vi "Main.vi"(11 "Module Admin":refnum<class "Delacor_lib_QMH_Cloneable Module Admin.lvclass">) -> ()   [LabVIEW 2023, in "Graph_data_collector.lvlib" / "Graph_UI.lvlib"]
doc: "This template is based off of the Queued Message Handler design pattern and the Queued Message Handler project template that ships with LabVIEW.\n\nThe main difference is that the queue is private to this module and communication between modules is performed via Broadcast and Request events.\n\nRequest events are wrapped in public API methods and are handled in the Event Handling Loop (EHL) of this VI. Any module can register for Broadcast events sent by this module. The EHL generates messages based on user interface actions.\n\nThe Message Handling Loop (MHL) processes messages generated by the EHL, or by other messages. The messages are string values, so new messages can be added easily to the Message Cases case structure in the MHL. Each message cluster can also provide an optional value for Message Data, which is a variant that can be converted to whatever message-specific data is required.\n_____\nBased on DQMH Project Template 6.1.0.94."
uses:
  Graph_UI.lvlib
  <vilib>/Delacor/Delacor QMH/Libraries/Cloneable Module Admin_class/Delacor_lib_QMH_Cloneable Module Admin.lvclass
  C:/Program Files/National Instruments/LabVIEW 2023/vi.lib/Delacor/Delacor QMH/Libraries/Module Admin_class/Delacor_lib_QMH_Module Admin.lvclass
  Module Data--cluster.ctl
  Data Control.ctl
  <vilib>/Delacor/Delacor QMH/Libraries/Message Queue_class/Delacor_lib_QMH_Message Queue.lvclass/Delacor_lib_QMH_Message Queue.ctl
  <vilib>/Delacor/Delacor QMH/Libraries/Cloneable Module Admin_class/Delacor_lib_QMH_Cloneable Module Admin.lvclass/Delacor_lib_QMH_Cloneable Module Admin.ctl
  Stop Argument--cluster.ctl
  New Data Argument--cluster.ctl
  SetP Argument--cluster.ctl
  <vilib>/Utility/miscctls.llb/LVPointTypeDef.ctl
  <vilib>/Delacor/Delacor QMH/Libraries/Module Admin_class/Delacor_lib_QMH_Module Admin.lvclass/Delacor_lib_QMH_Module Admin.ctl
  <vilib>/Delacor/Delacor QMH/Libraries/Message Queue_class/Delacor_lib_QMH_Enqueue Message (Single).vi
  <vilib>/Delacor/Delacor QMH/Libraries/Cloneable Module Admin_class/Delacor_lib_QMH_Get Module ID.vi
  <vilib>/Delacor/Delacor QMH/Libraries/Module Admin_class/Delacor_lib_QMH_Get External Launch.vi
  <vilib>/Utility/error.llb/Error Cluster From Error Code.vi
  <vilib>/ErrorRing/Error Ring.xnode
  <vilib>/Delacor/Delacor QMH/Libraries/Message Queue_class/Delacor_lib_QMH_Message Queue.lvclass
  Graph_data_collector.lvlib
panel:
  out "Общая ось":bool
  out "Персональные оси":bool
  in  "Оси":bool
  in  "Clear_Graph":bool
  out "error out":errorcluster
  out "Status":string
  in  "Simulate EHL Error":bool
  in  "Simulate MHL Error":bool
  out "XY Graph Time":cluster{"Value":timestamp[], "Value":dbl[]}[](graph)
  out "XY Graph Other":cluster{"OX":dbl[], "OY":dbl[]}[](graph)
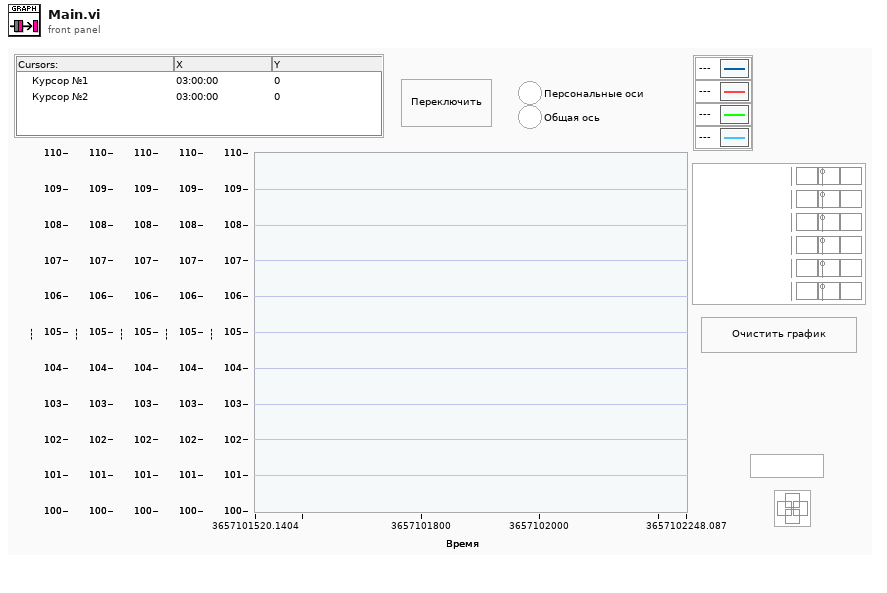
[diagram p1: front panel]
types:
  T1 = typedef "Graph_data_collector.lvlib/Graph_UI.lvlib/Module Data--cluster.ctl" = cluster{"Status":string, "XY Graph our ref":refnum<vi>, "Array Lable":string[], "Ось Y":i32[], "Ось Х":i32, "Graph size":i32, "appended array":T2[], "XY Graph ref":refnum<vi>}
  T2 = typedef "Graph_data_collector.lvlib/Data Control.ctl" = cluster{"Время":dbl, "Рпл1, МПа":dbl, "Vпл, см3":dbl, "Рпл2, МПа":dbl, "Ргор, МПа":dbl, "Ткд, градС":dbl, "R, Ом":dbl, "dL, мм":dbl, "Рэфф, МПа":dbl, "Рдм, МПа":dbl, "Q, мл":dbl, "Тнагр, градС":dbl, "ЦАП, градС":dbl}
  T3 = typedef "Graph_data_collector.lvlib/Graph_UI.lvlib/Request Events--cluster.ctl" = cluster{"Stop Module":refnum<user-event>, "Show Panel":refnum<user-event>, "Hide Panel":refnum<user-event>, "Show Diagram":refnum<user-event>, "Get Module Execution Status":refnum<user-event>, "New Data":refnum<user-event>, "SetP":refnum<user-event>}
  T4 = enum32{"invalid lock state", "Not Locked", "Locked (No Password)", "Password-protected"}
  T5 = typedef "Graph_data_collector.lvlib/Graph_UI.lvlib/Stop Argument--cluster.ctl" = cluster{"Module ID":i32, "Origin":string, "Exit via Stop Module Req?":bool, "Wait for Module to stop?":bool}
  T6 = typedef "Graph_data_collector.lvlib/Graph_UI.lvlib/New Data Argument--cluster.ctl" = cluster{"Module ID":i32, "Data":T2}
  T7 = typedef "Graph_data_collector.lvlib/Graph_UI.lvlib/SetP Argument--cluster.ctl" = cluster{"Module ID":i32, "Module Data":T1}
  T8 = typedef "LVPointTypeDef.ctl" = cluster{"Horizontal":i16, "Vertical":i16}
  T9 = enum32{"Invalid", "Standard", "Closed", "Hidden", "Minimized", "Maximized"}
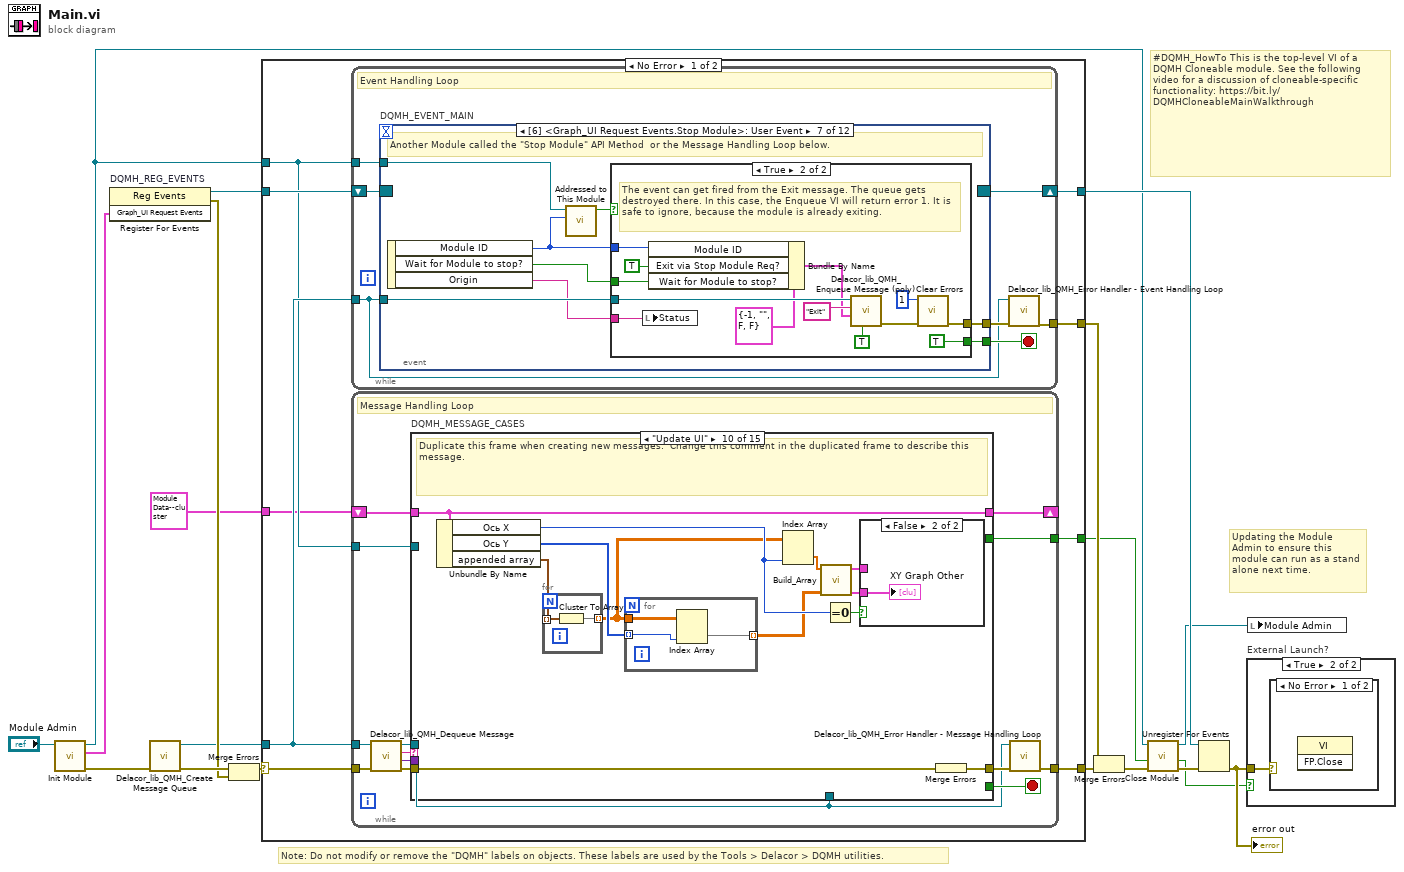
[diagram p0: block diagram]
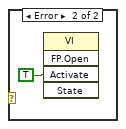
[diagram p3: hidden frame]
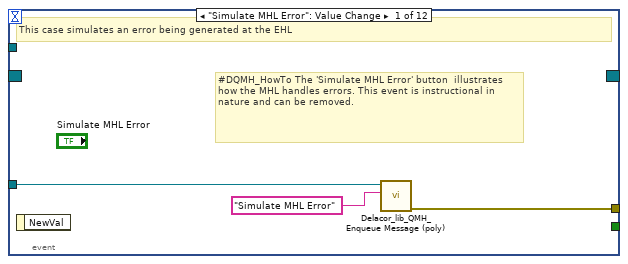
[diagram p4: hidden frame]
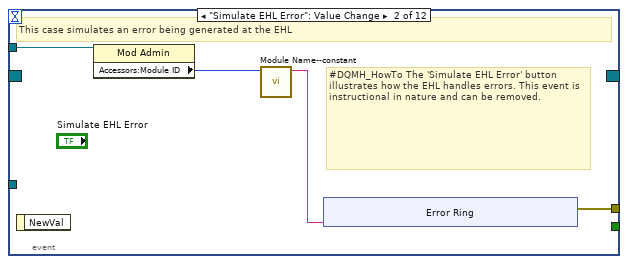
[diagram p5: hidden frame]
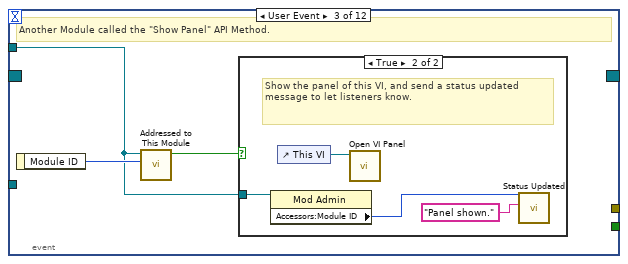
[diagram p6: hidden frame]
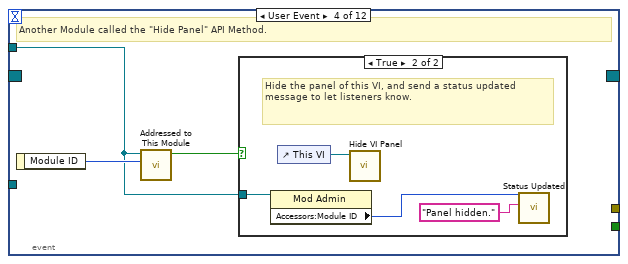
[diagram p8: hidden frame]
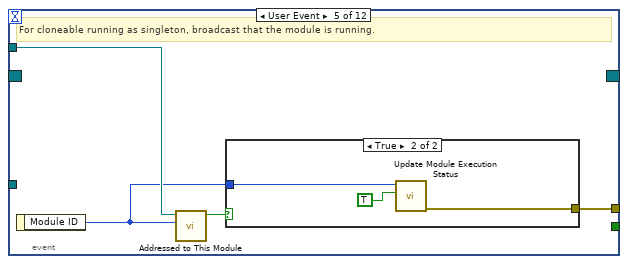
[diagram p10: hidden frame]
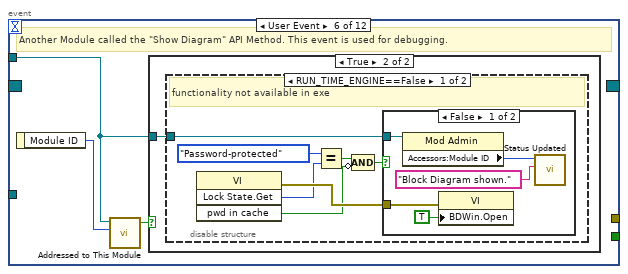
[diagram p12: hidden frame]
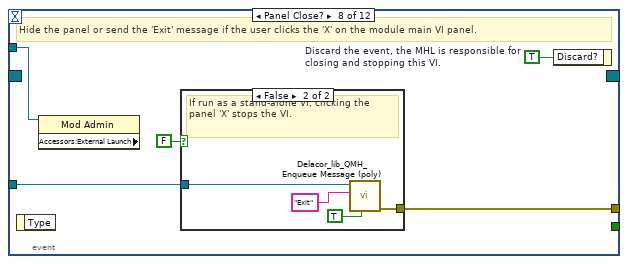
[diagram p17: hidden frame]
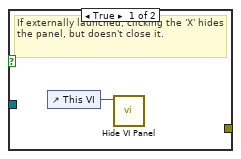
[diagram p18: hidden frame]
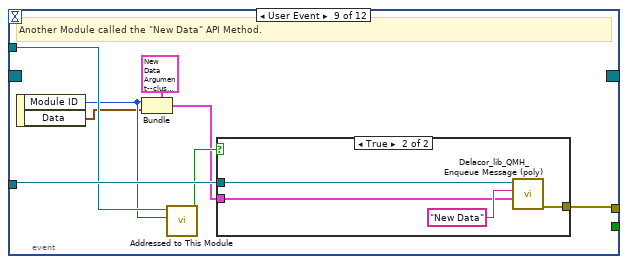
[diagram p19: hidden frame]
diagram:
  # "#DQMH_HowTo This is the top-level VI of a DQMH Cloneable module. See the following video for a discussion of cloneable-specific functionality: https://bit.ly/DQMHCloneableMainWalkthrough"
  # "Note: Do not modify or remove the \"DQMH\" labels on objects. These labels are used by the Tools > Delacor > DQMH utilities."
  # "Updating the Module Admin to ensure this module can run as a stand alone next time."
  n1 = call "Init Module.vi"("Cloneable Module Admin in"="Module Admin") -> ("error out"=w16:errorcluster, "Graph_UI Request Events"=w8:T3, "Cloneable Module Admin out"=w5:refnum<class "Delacor_lib_QMH_Cloneable Module Admin.lvclass">)  [unwired: 8 in]
  n2 = register-events "DQMH_REG_EVENTS"(w8) -> (reference out=w9:refnum<event-registration>, error out=w11:errorcluster)  [unwired: 2 in]
  n3 = call <vilib>:"Delacor_lib_QMH_Create Message Queue.vi"("error in"=w16) -> ("error out"=w13:errorcluster, "Message Queue"=w7:refnum<class "Delacor_lib_QMH_Message Queue.lvclass">)  [unwired: 9 in]
  n4 = Merge Errors(w13, w11) -> (w12:errorcluster)
  n5 = case shown="No Error" w12 {
    selector: w12 -> [w26 w356]
    tunnel: [w28 w355] -> w17
    tunnel: [w25 w363] -> w10
    tunnel: w9 -> [w24 w363]
    tunnel: w7 -> [w23 w354]
    tunnel: [w27 _] -> w18
    tunnel: w5 -> [w22 w359]
    tunnel: [w21 _] -> w3
    tunnel: T1 {"Status"="", "XY Graph our ref"=refnum, "Array Lable"=[], "Ось Y"=[], "Ось Х"=0, "Graph size"=20000, "appended array"=[], "XY Graph ref"=refnum} ("Data Cluster") -> [w20 _]
    frame No Error {
      n6 = while {
        tunnel: w23 -> [w29]
        shift-right: [w32] -> w25
        shift-left: w24 -> [w33]
        tunnel: [w34] -> w27
        tunnel: w22 -> [w30]
        stop <- w31 stop-if-true
        # "Event Handling Loop"
        n7 = event "DQMH_EVENT_MAIN" shown="[6] <Graph_UI Request Events.Stop Module>: User Event" {
          selector: w33 -> [_ _ _ _ _ _ _ _ _ _ _ _]
          dyn-events: [_ _ _ _ _ _ _ _ _ _ _ _] -> w32
          timeout: _ -> [_ _ _ _ _ _ _ _ _ _ _ _]
          tunnel: [_ _ _ _ _ _ w90 _ _ _ _ _] -> w31
          tunnel: w29 -> [w37 _ _ _ _ _ w93 w109 w125 w131 w140 w146]
          tunnel: [w38 w42 _ _ w67 _ w94 w112 w118 w130 w133 w145] -> w35
          tunnel: w30 -> [_ w41 w50 w57 w65 w71 w92 w110 w123 _ w138 _]
          event "Simulate MHL Error": Value Change {
            # "#DQMH_HowTo The 'Simulate MHL Error' button  illustrates how the MHL handles errors. This event is instructional in nature and can be removed."
            # "This case simulates an error being generated at the EHL"
            n8 = event-data() -> ()  [unwired: 1 in, 1 out]
            n9 = call-poly <vilib>:"Delacor_lib_QMH_Enqueue Message (poly).vi"("Message"="Simulate MHL Error", "Message Queue in"=w37) -> ("error out"=w38:errorcluster)  [unwired: 8 in, 1 out]
          }
          event "Simulate EHL Error": Value Change {
            # "#DQMH_HowTo The 'Simulate EHL Error' button  illustrates how the EHL handles errors. This event is instructional in nature and can be removed."
            # "This case simulates an error being generated at the EHL"
            n10 = event-data() -> ()  [unwired: 1 in, 1 out]
            n11 = property class="Mod Admin"(reference=w41) -> ("Accessors:Module ID"=w40:i32)  [unwired: 1 in, 2 out]
            n12 = call "Module Name--constant.vi"("Module ID"=w40) -> ("Module Name"=w39:string)  [unwired: 10 in]
            n13 = xnode "Error Ring"("parameter 0"=w39) -> ("error out"=w42:errorcluster)
          }
          event User Event {
            # "Another Module called the \"Show Panel\" API Method."
            n14 = event-data() -> ("Module ID"=w51:i32)  [unwired: 1 in]
            n15 = call "Addressed to This Module.vi"("Module ID from Argument"=w51, "Module Admin"=w50) -> ("Addressed to this instance?"=w52:bool)  [unwired: 8 in, 1 out]
            n16 = case shown="True" w52 {
              tunnel: w50 -> [_ w54]
              frame False {
              }
              frame True {
                # "Show the panel of this VI, and send a status updated message to let listeners know."
                n17 = property class="Mod Admin"(reference=w54) -> ("Accessors:Module ID"=w53:i32)  [unwired: 1 in, 2 out]
                n18 = control-ref of="This VI"() -> (w56:refnum<vi>)
                n19 = call "Open VI Panel.vi"("VI"=w56) -> ()  [unwired: 10 in, 1 out]
                n20 = call "Status Updated.vi"("Status"="Panel shown." ("format string"), "Module ID"=w53) -> ()  [unwired: 9 in, 1 out]
              }
            }
          }
          event User Event {
            # "Another Module called the \"Hide Panel\" API Method."
            n21 = event-data() -> ("Module ID"=w58:i32)  [unwired: 1 in]
            n22 = call "Addressed to This Module.vi"("Module ID from Argument"=w58, "Module Admin"=w57) -> ("Addressed to this instance?"=w59:bool)  [unwired: 8 in, 1 out]
            n23 = case shown="True" w59 {
              tunnel: w57 -> [_ w61]
              frame False {
              }
              frame True {
                # "Hide the panel of this VI, and send a status updated message to let listeners know."
                n24 = property class="Mod Admin"(reference=w61) -> ("Accessors:Module ID"=w60:i32)  [unwired: 1 in, 2 out]
                n25 = control-ref of="This VI"() -> (w63:refnum<vi>)
                n26 = call "Hide VI Panel.vi"("VI"=w63) -> ()  [unwired: 10 in, 1 out]
                n27 = call "Status Updated.vi"("Status"="Panel hidden." ("format string"), "Module ID"=w60) -> ()  [unwired: 9 in, 1 out]
              }
            }
          }
          event User Event {
            # "For cloneable running as singleton, broadcast that the module is running."
            n28 = event-data() -> ("Module ID"=w64:i32)  [unwired: 1 in]
            n29 = call "Addressed to This Module.vi"("Module ID from Argument"=w64, "Module Admin"=w65) -> ("Addressed to this instance?"=w66:bool)  [unwired: 8 in, 1 out]
            n30 = case shown="True" w66 {
              tunnel: [_ w70] -> w67
              tunnel: w64 -> [_ w69]
              frame False {
              }
              frame True {
                n31 = call "Update Module Execution Status.vi"("Running?"=TRUE, "Module ID"=w69) -> ("error out"=w70:errorcluster)  [unwired: 9 in]
              }
            }
          }
          event User Event {
            # "Another Module called the \"Show Diagram\" API Method. This event is used for debugging."
            n32 = event-data() -> ("Module ID"=w72:i32)  [unwired: 1 in]
            n33 = call "Addressed to This Module.vi"("Module ID from Argument"=w72, "Module Admin"=w71) -> ("Addressed to this instance?"=w73:bool)  [unwired: 8 in, 1 out]
            n34 = case shown="True" w73 {
              tunnel: w71 -> [_ w74]
              frame False {
              }
              frame True {
                n35 = disable-structure shown="RUN_TIME_ENGINE==False" {
                  disable-tunnel: w74 -> [w75 _]
                  frame condition #0 (active) {
                    # "functionality not available in exe"
                    n36 = invoke class="VI" method="Lock State.Get"() -> (error out=w81:errorcluster, "Get Lock State"=w80:T4, "pwd in cache"=w77:bool)  [unwired: 4 in, 1 out]
                    n37 = Equal?(x=T4."Password-protected", y=w80) -> (x = y?=w78:bool)
                    n38 = Compound Arithmetic op=AND(w78, invert w77) -> (w76:bool)
                    n39 = case shown="False" w76 {
                      tunnel: w81 -> [w86 _]
                      tunnel: w75 -> [w83 _]
                      frame False {
                        n40 = property class="Mod Admin"(reference=w83) -> ("Accessors:Module ID"=w82:i32)  [unwired: 1 in, 2 out]
                        n41 = property class="VI"(error in=w86, "BDWin.Open"=TRUE ("Block Diagram Window:Open")) -> ()  [unwired: 1 in, 2 out]
                        n42 = call "Status Updated.vi"("Status"="Block Diagram shown." ("format string"), "Module ID"=w82) -> ()  [unwired: 9 in, 1 out]
                      }
                      frame True {
                        # "Password-protected VI, and the password is not in the cache. Do not show the diagram."
                      }
                    }
                  }
                  frame condition #1 {
                  }
                }
              }
            }
          }
          event User Event {
            # "Another Module called the \"Stop Module\" API Method  or the Message Handling Loop below."
            n43 = event-data() -> ("Module ID"=w88:i32, "Wait for Module to stop?"=w89:bool, "Origin"=w87:string)  [unwired: 1 in]
            n44 = call "Addressed to This Module.vi"("Module ID from Argument"=w88, "Module Admin"=w92) -> ("Addressed to this instance?"=w91:bool)  [unwired: 8 in, 1 out]
            n45 = case shown="True" w91 {
              tunnel: [_ w106] -> w94
              tunnel: w93 -> [_ w102]
              tunnel: [_ TRUE] -> w90
              tunnel: w89 -> [_ w97]
              tunnel: w88 -> [_ w99]
              tunnel: w87 -> [_ w95]
              frame False {
              }
              frame True {
                # "The event can get fired from the Exit message. The queue gets destroyed there. In this case, the Enqueue VI will return error 1. It is safe to ignore, because the module is already exiting."
                n46 = local write "Status"(w95) -> ()
                n47 = Bundle By Name(cluster=T5 {"Module ID"=-1, "Origin"="", "Exit via Stop Module Req?"=FALSE, "Wait for Module to stop?"=FALSE} ("Stop Argument"), "Module ID"=w99, "Exit via Stop Module Req?"=TRUE, "Wait for Module to stop?"=w97) -> (w96:T5)
                n48 = call-poly <vilib>:"Delacor_lib_QMH_Enqueue Message (poly).vi"("Priority Message? (F)"=TRUE, "Message Data"=w96, "Message"="Exit", "Message Queue in"=w102) -> ("error out"=w107:errorcluster)  [unwired: 6 in, 1 out]
                n49 = call <vilib>:"Clear Errors.vi"("error in (no error)"=w107, "specific error code to clear (0: all)"=1) -> ("error out"=w106:errorcluster)  [unwired: 4 in, 1 out]
              }
            }
          }
          event Panel Close? {
            w111 = TRUE  # Discard the event, the MHL is responsible for closing and stopping this VI.
            # "Hide the panel or send the 'Exit' message if the user clicks the 'X' on the module main VI panel."
            n50 = event-data() -> ()  [unwired: 1 in, 1 out]
            n51 = property class="Mod Admin" props=["Accessors:External Launch"](reference=w110) -> ()  [unwired: 1 in, 3 out]
            n52 = case shown="False" FALSE {
              tunnel: w109 -> [_ w116]
              tunnel: [_ w117] -> w112
              frame True {
                # "If externally launched, clicking the 'X' hides the panel, but doesn't close it."
                n53 = control-ref of="This VI"() -> (w113:refnum<vi>)
                n54 = call "Hide VI Panel.vi"("VI"=w113) -> ()  [unwired: 10 in, 1 out]
              }
              frame False {
                # "If run as a stand-alone VI, clicking the panel 'X' stops the VI."
                n55 = call-poly <vilib>:"Delacor_lib_QMH_Enqueue Message (poly).vi"("Priority Message? (F)"=TRUE, "Message"="Exit", "Message Queue in"=w116) -> ("error out"=w117:errorcluster)  [unwired: 7 in, 1 out]
              }
            }
            n56 = event-data("Discard?"=w111) -> ()  [unwired: 1 in, 1 out]
          }
          event User Event {
            # "Another Module called the \"New Data\" API Method."
            n57 = event-data() -> ("Module ID"=w120:i32, "Data"=w119:T2)  [unwired: 1 in]
            n58 = Bundle(cluster=T6 {"Module ID"=-1, "Data"={"Время"=0.0, "Рпл1, МПа"=0.0, "Vпл, см3"=0.0, "Рпл2, МПа"=0.0, "Ргор, МПа"=0.0, "Ткд, градС"=0.0, "R, Ом"=0.0, "dL, мм"=0.0, "Рэфф, МПа"=0.0, "Рдм, МПа"=0.0, "Q, мл"=0.0, "Тнагр, градС"=0.0, "ЦАП, градС"=0.0}} ("New Data Argument"), "Module ID"=w120, "Data"=w119) -> (w121:T6)
            n59 = call "Addressed to This Module.vi"("Module ID from Argument"=w120, "Module Admin"=w123) -> ("Addressed to this instance?"=w124:bool)  [unwired: 8 in, 1 out]
            n60 = case shown="True" w124 {
              tunnel: w125 -> [_ w129]
              tunnel: w121 -> [_ w127]
              tunnel: [_ w126] -> w118
              frame False {
              }
              frame True {
                n61 = call-poly <vilib>:"Delacor_lib_QMH_Enqueue Message (poly).vi"("Message Data"=w127, "Message"="New Data", "Message Queue in"=w129) -> ("error out"=w126:errorcluster)  [unwired: 7 in, 1 out]
              }
            }
          }
          event "Clear_Graph": Value Change {
            n62 = event-data() -> ()  [unwired: 1 in, 1 out]
            n63 = call-poly <vilib>:"Delacor_lib_QMH_Enqueue Message (poly).vi"("Message"="Clear", "Message Queue in"=w131) -> ("error out"=w130:errorcluster)  [unwired: 8 in, 1 out]
          }
          event User Event {
            # "Another Module called the \"SetP\" API Method."
            n64 = event-data() -> ("Module ID"=w135:i32, "Module Data"=w134:T1)  [unwired: 1 in]
            n65 = Bundle(cluster=T7 {"Module ID"=-1, "Module Data"={"Status"="", "XY Graph our ref"=refnum, "Array Lable"=[], "Ось Y"=[], "Ось Х"=0, "Graph size"=20000, "appended array"=[], "XY Graph ref"=refnum}} ("SetP Argument"), "Module ID"=w135, "Module Data"=w134) -> (w136:T7)
            n66 = call "Addressed to This Module.vi"("Module ID from Argument"=w135, "Module Admin"=w138) -> ("Addressed to this instance?"=w139:bool)  [unwired: 8 in, 1 out]
            n67 = case shown="True" w139 {
              tunnel: w140 -> [_ w144]
              tunnel: w136 -> [_ w142]
              tunnel: [_ w141] -> w133
              frame False {
              }
              frame True {
                n68 = call-poly <vilib>:"Delacor_lib_QMH_Enqueue Message (poly).vi"("Message Data"=w142, "Message"="SetP", "Message Queue in"=w144) -> ("error out"=w141:errorcluster)  [unwired: 7 in, 1 out]
              }
            }
          }
          event "Оси": Value Change {
            n69 = event-data() -> ()  [unwired: 1 in, 3 out]
            n70 = call-poly <vilib>:"Delacor_lib_QMH_Enqueue Message (poly).vi"("Message"="Change_OY", "Message Queue in"=w146) -> ("error out"=w145:errorcluster)  [unwired: 8 in, 1 out]
          }
        }
        n71 = call-dynamic "Delacor_lib_QMH_Error Handler - Event Handling Loop.vi"("error in"=w35, "Message Queue in"=w29) -> ("dup error in"=w34:errorcluster)  [unwired: 8 in, 1 out]
      }
      n72 = while {
        tunnel: w23 -> [w151]
        shift-right: [w155] -> _
        shift-left: w20 -> [w156]
        tunnel: w26 -> [w159]
        tunnel: [w157] -> w28
        tunnel: w22 -> [w150]
        tunnel: [w149] -> w21
        stop <- w154 stop-if-true
        # "Message Handling Loop"
        n73 = call-dynamic "Delacor_lib_QMH_Dequeue Message.vi"("error in"=w159, "Message Queue in"=w151) -> ("error out"=w158:errorcluster, "Message Data"=w152:variant, "Message"=w153:string, "Message Queue out"=w148:refnum<class "Delacor_lib_QMH_Message Queue.lvclass">)  [unwired: 6 in]
        n74 = case "DQMH_MESSAGE_CASES" shown="\"Update UI\"" w153 {
          selector: w153 -> [_ _ _ _ _ _ _ _ _ _ _ _ _ _ w341]
          tunnel: w148 -> [_ _ _ w205 _ w218 w240 _ _ _ _ w292 _ w331 _]
          tunnel: w158 -> [w180 w184 w204 w213 w216 w224 w244 w249 w267 w281 w290 w301 w314 w337 w343]
          tunnel: [w179 w184 w194 w207 w215 w227 w243 w248 w266 w280 w290 w297 w313 w334 w344] -> w160
          tunnel: w156 -> [w172 w183 w190 _ w214 w226 w242 w247 w262 w279 w289 w296 w311 w330 w342]
          tunnel: [w171 w183 w186 w209 w214 w226 w242 w246 w255 w279 w289 w296 w311 w330 w342] -> w155
          tunnel: [_ _ _ _ _ _ _ _ _ _ _ _ _ w329 _] -> w154
          tunnel: w152 -> [_ _ w203 w212 _ w223 _ _ _ _ _ w295 _ w327 _]
          tunnel: w150 -> [w166 _ _ _ _ _ _ _ w261 _ _ w294 w309 w323 w339]
          tunnel: [_ _ _ _ _ _ _ _ _ _ _ _ _ w325 _] -> w149
          tunnel: w148 -> [_ _ w192 _ _ _ _ _ _ _ _ _ _ _ _]
          frame "Initialize" {
            w163 = "Initial Message" ("Initial Message")
            # "Initialize - Any operation that needs to be done before the module can receive messages. Synchronize Caller Events.vi will inform Start Module.vi that the module has launched and is ready to receive messages. Module Did Init.vi will broadcast that the module initialized."
            n75 = call "Synchronize Caller Events.vi"("error in (no error)"=w180, "Module Admin"=w166) -> ("error out"=w162:errorcluster, "Module Admin out"=w165:refnum<class "Delacor_lib_QMH_Cloneable Module Admin.lvclass">)  [unwired: 8 in]
            n76 = property class="Mod Admin"(reference=w165) -> ("Accessors:Module ID"=w168:i32, "Accessors:External Launch"=w167:bool)  [unwired: 1 in, 2 out]
            n77 = call "Module Name--constant.vi"("Module ID"=w168) -> ("Module Name"=w176:string)  [unwired: 10 in]
            n78 = property class="VI"("Front Panel.Title"=w176) -> (reference out=w178:refnum<vi>, error out=w182:errorcluster)  [unwired: 2 in]
            n79 = Select(t=T9."Hidden" ("State"), s=w167, f=T9."Standard" ("State")) -> (s? t:f=w173:T9)
            n80 = invoke class="VI" method="FP.Open"(reference=w178, error in=w182, "State"=w173) -> (reference out=w177:refnum<vi>, error out=w181:errorcluster)  [unwired: 2 in, 3 out]
            n81 = Bundle By Name(cluster=w172, "Graph size"=20000, "Status"=w163) -> (w171:T1)
            n82 = call "Module Name--constant.vi"("Module ID"=w168) -> ("Module Name"=w169:string)  [unwired: 10 in]
            n83 = invoke class="VI" method="FP.Center"(reference=w177, error in=w181) -> ()  [unwired: 1 in, 3 out]
            n84 = property on="Pane" class="Pane"("Origin"=T8 {"Horizontal"=0, "Vertical"=0}) -> ()  [unwired: 2 in, 2 out]
            n85 = call "Module Did Init.vi"("error in (no error)"=w162, "Initialized?"=TRUE, "Origin"=w169, "Module ID"=w168) -> ("error out"=w179:errorcluster)  [unwired: 7 in]
            "Status" <- w163
          }
          frame "---Module Specific---" {
            # "Separator -- The following cases handle messages specific to this Module."
          }
          frame "New Data" {
            n86 = Unbundle By Name(w190) -> ("Graph size"=w189:i32, "appended array"=w187:T2[])
            n87 = Variant To Data(error in=w204, type=T6 {"Module ID"=-1, "Data"={"Время"=0.0, "Рпл1, МПа"=0.0, "Vпл, см3"=0.0, "Рпл2, МПа"=0.0, "Ргор, МПа"=0.0, "Ткд, градС"=0.0, "R, Ом"=0.0, "dL, мм"=0.0, "Рэфф, МПа"=0.0, "Рдм, МПа"=0.0, "Q, мл"=0.0, "Тнагр, градС"=0.0, "ЦАП, градС"=0.0}} ("New Data Argument"), Variant=w203) -> (data=w201:T6, error out=w193:errorcluster)
            n88 = Unbundle By Name(w201) -> ("Data"=w188:T2)
            n89 = Build Array (concatenate)(w187, w188) -> (w195:T2[])
            n90 = Array Size(array=w195) -> (size(s)=w198:i32)
            n91 = Subtract(x=w198, y=w189) -> (x-y=w200:i32)
            n92 = Decrement(x=w198) -> (x-1=w199:i32)
            n93 = Greater Or Equal?(x=w199, y=w189) -> (x >= y?=w196:bool)
            n94 = Delete From Array(array=w195, length=w189, index=w200) -> (deleted portion=w197:T2[])  [unwired: 1 out]
            n95 = Select(t=w197, s=w196, f=w195) -> (s? t:f=w185:T2[])
            n96 = Bundle By Name(cluster=w190, "appended array"=w185) -> (w186:T1)
            n97 = call-poly <vilib>:"Delacor_lib_QMH_Enqueue Message (poly).vi"("error in"=w193, "Message Data"=w188, "Message"="Update UI", "Message Queue in"=w192) -> ("error out"=w194:errorcluster)  [unwired: 6 in, 1 out]
          }
          frame "SetP" {
            n98 = Variant To Data(error in=w213, type=T7 {"Module ID"=-1, "Module Data"={"Status"="", "XY Graph our ref"=refnum, "Array Lable"=[], "Ось Y"=[], "Ось Х"=0, "Graph size"=20000, "appended array"=[], "XY Graph ref"=refnum}} ("SetP Argument"), Variant=w212) -> (data=w210:T7, error out=w206:errorcluster)
            n99 = Unbundle By Name(w210) -> ("Module Data"=w209:T1)  [unwired: 1 out]
            n100 = call-poly <vilib>:"Delacor_lib_QMH_Enqueue Message (poly).vi"("error in"=w206, "Message"="Init UI", "Message Queue in"=w205) -> ("error out"=w207:errorcluster)  [unwired: 7 in, 1 out]
          }
          frame "---Copy This Frame---" {
            # "Duplicate this frame when creating new messages.  Change this comment in the duplicated frame to describe this message."
            n101 = Merge Errors(w216) -> (w215:errorcluster)
          }
          frame "Update_OY" {
            # "Duplicate this frame when creating new messages.  Change this comment in the duplicated frame to describe this message."
            n102 = Unbundle By Name(w226) -> ("XY Graph ref"=w225:refnum<vi>, "Ось Y"=w217:i32[])
            n103 = Variant To Data(error in=w224, type=u32 0 ("number"), Variant=w223) -> (data=w221:u32, error out=w220:errorcluster)
            n104 = case shown="2" w221 {
              tunnel: w225 -> [_ w234]
              tunnel: w220 -> [w230 _]
              tunnel: [w229 w233] -> w219
              tunnel: w218 -> [w228 _]
              tunnel: w217 -> [_ w232]
              frame 1, Default {
                n105 = call-poly <vilib>:"Delacor_lib_QMH_Enqueue Message (poly).vi"("error in"=w230, "Message"="Init UI", "Message Queue in"=w228) -> ("error out"=w229:errorcluster)  [unwired: 7 in, 1 out]
              }
              frame 2 {
                n106 = call "Lock_1_Plot.vi"("Ось Y"=w232, "XY Graph ref"=w234) -> ("error out"=w233:errorcluster)  [unwired: 9 in]
              }
            }
            n107 = Merge Errors(w219, w220) -> (w227:errorcluster)
          }
          frame "Change_OY" {
            # "Duplicate this frame when creating new messages.  Change this comment in the duplicated frame to describe this message."
            n108 = local read "Персональные оси"() -> (w237:bool)
            n109 = Not(x=w237) -> (.not. x?=w238:bool)
            n110 = local write "Персональные оси"(w238) -> ()
            n111 = local write "Общая ось"(w237) -> ()
            n112 = Build Array(w238, w237) -> (w236:bool[])
            n113 = Boolean Array To Number(Boolean array=w236) -> (number=w235:u32)
            n114 = call-poly <vilib>:"Delacor_lib_QMH_Enqueue Message (poly).vi"("Message Data"=w235, "Message"="Update_OY", "Message Queue in"=w240) -> ("error out"=w239:errorcluster)  [unwired: 7 in, 1 out]
            n115 = Merge Errors(w239, w244) -> (w243:errorcluster)
          }
          frame "Clear" {
            # "Duplicate this frame when creating new messages.  Change this comment in the duplicated frame to describe this message."
            n116 = Bundle By Name(cluster=w247, "appended array"=T2[] []) -> (w246:T1)
            n117 = Merge Errors(w249) -> (w248:errorcluster)
          }
          frame "Init UI" {
            # "Duplicate this frame when creating new messages.  Change this comment in the duplicated frame to describe this message."
            n118 = property class="Mod Admin"(reference=w261) -> (error out=w257:errorcluster, "Accessors:Module ID"=w260:i32)  [unwired: 1 in, 1 out]
            n119 = Unbundle By Name(w262) -> ("Array Lable"=w263:string[], "Ось Y"=w251:i32[], "Ось Х"=w264:i32)
            n120 = control-ref of="XY Graph Time"() -> (w265:refnum<vi>)
            n121 = Array Size(array=w251) -> (size(s)=w250:i32)
            n122 = control-ref of="XY Graph Other"() -> (w256:refnum<vi>)
            n123 = call "Init UI XY Graph.vi"("XY Graph Other"=w256, "Ось Y"=w251, "Ось Х"=w264, "Array Lable"=w263, "XY Graph Time in ref"=w265) -> ("error out"=w259:errorcluster, "XY Graph ref"=w252:refnum<vi>)  [unwired: 5 in]
            n124 = for {
              N: w250 -> [_]
              tunnel: w252 -> [w269]
              i -> [w268]
              n125 = property on="Property Node" class="XYGraph"(reference=w269, "Active Plot"=w268, "Plot.YScaleIdx"=w268) -> ()  [unwired: 1 in, 2 out]
            }
            n126 = call "Show Panel.vi"("error in (no error)"=w259, "Module ID"=w260) -> ("error out"=w258:errorcluster)  [unwired: 9 in]
            n127 = Bundle By Name(cluster=w262, "XY Graph ref"=w252) -> (w255:T1)
            n128 = Merge Errors(w258, w257, w267) -> (w266:errorcluster)
            "Персональные оси" <- TRUE ("Персональные оси")
            "Общая ось" <- FALSE ("Общая ось")
          }
          frame "Update UI" {
            # "Duplicate this frame when creating new messages.  Change this comment in the duplicated frame to describe this message."
            n129 = Unbundle By Name(w279) -> ("Ось Х"=w277:i32, "Ось Y"=w278:i32[], "appended array"=w270:T2[])
            n130 = for {
              tunnel: w270 -> [w285] mode=indexing
              tunnel: [w284] -> w276 mode=indexing
              n131 = Cluster To Array(cluster=w285) -> (array=w284:dbl[])
            }
            n132 = for {
              tunnel: w278 -> [w288] mode=indexing
              tunnel: [w287] -> w274 mode=indexing
              tunnel: w276 -> [w286]
              n133 = Index Array(array=w286, index (col)=w288) -> (element=w287:dbl[])  [unwired: 1 in]
            }
            n134 = Index Array(array=w276, index (col)=w277) -> (element=w273:dbl[])  [unwired: 1 in]
            n135 = call "Build_Array.vi"("OY"=w274, "OX"=w273) -> ("Other"=w272:cluster{"OX":dbl[], "OY":dbl[]}[], "Time"=w271:cluster{timestamp[], "OY":dbl[]}[])  [unwired: 8 in]
            n136 = Equal To 0?(x=w277) -> (x = 0?=w275:bool)
            n137 = case shown="False" w275 {
              tunnel: w272 -> [_ w283]
              tunnel: w271 -> [w282 _]
              frame True {
                "XY Graph Time" <- w282
              }
              frame False {
                "XY Graph Other" <- w283
              }
            }
            n138 = Merge Errors(w281) -> (w280:errorcluster)
          }
          frame "---Exit and Error Handling---" {
            # "Separator - the following cases handle errors and exit messages."
          }
          frame "Error" {
            # "#CodeRecommended - If you ever change the name of this \"Error\" message, you'll need to update the name in the Check Loop Error.vi as well."
            # "#CodeRecommended - If the module is running in standalone mode (External Launch = FALSE), this code will pop up an error dialog and call the 'Exit' message if an error occurs. Add more fine-grained error handling here."
            # "Error - Check the error message data and respond accordingly. This message is sent by the \"Error Handler\" VIs at the end of each loop in this application."
            n139 = property class="Mod Admin"(reference=w294) -> ("Accessors:External Launch"=w293:bool, "Accessors:Module ID"=w291:i32)  [unwired: 1 in, 2 out]
            n140 = Variant To Data(error in=w301, type=errorcluster {"status"=FALSE, "code"=0, "source"=""} ("error constant"), Variant=w295) -> (data=w302:errorcluster, error out=w299:errorcluster)
            n141 = call "Error Reported.vi"("Error"=w302, "Module ID"=w291) -> ()  [unwired: 9 in, 1 out]
            n142 = case shown="False" w293 {
              tunnel: [w307 _] -> w298
              tunnel: w292 -> [w305 _]
              tunnel: w302 -> [w306 _]
              frame False {
                # "If the module is running standalone, then pop up an error dialog and call the \"Exit\" message."
                n143 = call <vilib>:"Simple Error Handler.vi"("error in (no error)"=w306) -> ()  [unwired: 4 in, 5 out]
                n144 = call-poly <vilib>:"Delacor_lib_QMH_Enqueue Message (poly).vi"("Priority Message? (F)"=TRUE, "Message"="Exit", "Message Queue in"=w305) -> ("error out"=w307:errorcluster)  [unwired: 7 in, 1 out]
              }
              frame True {
                # "If the module was launched externally, calling the Error Reported broadcast VI is the only action performed by the \"Error\" message. The module's caller can then process the error appropriately."
              }
            }
            n145 = Merge Errors(w299, w298) -> (w297:errorcluster)
            n146 = local write "error out"(w297) -> ()
          }
          frame "Simulate MHL Error" {
            # "#DQMH_HowTo The 'Simulate MHL Error' button  illustrates how the MHL handles errors. This event is instructional in nature and can be removed."
            # "Simulate an error occurring at the MHL"
            n147 = property class="Mod Admin"(reference=w309) -> ("Accessors:Module ID"=w310:i32)  [unwired: 1 in, 2 out]
            n148 = call "Module Name--constant.vi"("Module ID"=w310) -> ("Module Name"=w308:string)  [unwired: 10 in]
            n149 = xnode "Error Ring"("parameter 0"=w308) -> ("error out"=w312:errorcluster)
            n150 = Merge Errors(w314, w312) -> (w313:errorcluster)
          }
          frame "Exit" {
            w328 = 91  # 91: not all Exit messages will have an argument
            w329 = TRUE  # Stop the VI
            # "Release the message queue reference"
            # "Exit - Exit the application."
            n151 = Variant To Data(error in=w337, type=T5 {"Module ID"=-1, "Origin"="", "Exit via Stop Module Req?"=FALSE, "Wait for Module to stop?"=FALSE} ("Stop Argument"), Variant=w327) -> (data=w324:T5, error out=w332:errorcluster)
            n152 = call <vilib>:"Clear Errors.vi"("error in (no error)"=w332, "specific error code to clear (0: all)"=w328) -> ("error out"=w336:errorcluster)  [unwired: 4 in, 1 out]
            n153 = control-ref of="This VI"() -> (w322:refnum<vi>)
            n154 = call-dynamic "Delacor_lib_QMH_Release Message Queue.vi"("error in"=w336, "Message Queue"=w331) -> ("error out"=w335:errorcluster)  [unwired: 9 in]
            n155 = call "Handle Exit.vi"("Stop Argument"=w324, "Module Admin in"=w323, "VI reference"=w322) -> ("error out"=w333:errorcluster, "Wait for Stop?"=w325:bool)  [unwired: 7 in]
            n156 = Merge Errors(w335, w333) -> (w334:errorcluster)
          }
          frame Default {
            # "'Default' case only runs if there is a message that isn't defined in any of the other cases.  Output a programming error."
            n157 = property class="Mod Admin"(reference=w339) -> ("Accessors:Module ID"=w338:i32)  [unwired: 1 in, 2 out]
            n158 = call "Module Name--constant.vi"("Module ID"=w338) -> ("Module Name"=w340:string)  [unwired: 10 in]
            n159 = xnode "Error Ring"("parameter 0"=w341, "parameter 1"=w340) -> ("error out"=w345:errorcluster)
            n160 = Merge Errors(w343, w345) -> (w344:errorcluster)
          }
        }
        n161 = call-dynamic "Delacor_lib_QMH_Error Handler - Message Handling Loop.vi"("error in"=w160, "Message Queue in"=w148) -> ("dup error in"=w157:errorcluster)  [unwired: 8 in, 1 out]
      }
    }
    frame Error {
      n162 = call "Synchronize Caller Events.vi"("Module Admin"=w359) -> ("Module Admin out"=w358:refnum<class "Delacor_lib_QMH_Cloneable Module Admin.lvclass">)  [unwired: 9 in, 1 out]
      n163 = property class="Mod Admin"(reference=w358) -> ("Accessors:Module ID"=w357:i32)  [unwired: 1 in, 2 out]
      n164 = call-dynamic "Delacor_lib_QMH_Release Message Queue.vi"("error in"=w356, "Message Queue"=w354) -> ("error out"=w355:errorcluster)  [unwired: 9 in]
      n165 = call "Module Name--constant.vi"("Module ID"=w357) -> ("Module Name"=w362:string)  [unwired: 10 in]
      n166 = Format Into String(format string="An error occurred during initialization. %s is no longer running.", w362) -> (resulting string=w360:string)  [unwired: 2 in, 1 out]
      n167 = call "Error Reported.vi"("Additional Information"=w360, "Error"=w355, "Module ID"=w357) -> ()  [unwired: 8 in, 1 out]
    }
  }
  n168 = Merge Errors(w18, w17) -> (w19:errorcluster)
  n169 = call "Close Module.vi"("error in"=w19, "Wait for stop?"=w3, "Module Admin in"=w5) -> ("error out"=w15:errorcluster, "External Launch"=w2:bool, "Module Admin out"=w4:refnum<class "Delacor_lib_QMH_Cloneable Module Admin.lvclass">)  [unwired: 6 in]
  n170 = Unregister For Events(event registration refnum=w10, error in=w15) -> (error out=w14:errorcluster)
  "error out" <- w14
  n171 = case "External Launch?" shown="True" w2 {
    tunnel: w14 -> [_ w364]
    frame False {
    }
    frame True {
      n172 = case shown="No Error" w364 {
        frame No Error {
          n173 = invoke class="VI" method="FP.Close"() -> ()  [unwired: 3 in, 3 out]
        }
        frame Error {
          n174 = invoke class="VI" method="FP.Open"("Activate"=TRUE ("Activate?")) -> ()  [unwired: 4 in, 5 out]
        }
      }
    }
  }
  n175 = local write "Module Admin"(w4) -> ()
